vi "Set Controls State When Stopped.vi"(8 "error in (no error)":errorcluster, 11 "TS UI Data in":T1) -> (0 "error out":errorcluster)   [LabVIEW 2015]
uses:
  Type defs/TS UI Data.ctl
  Type defs/Nest cluster.ctl
panel:
  # "SCANNED DATA"
  # "ITAC DATA"
  # "DoIP DATA"
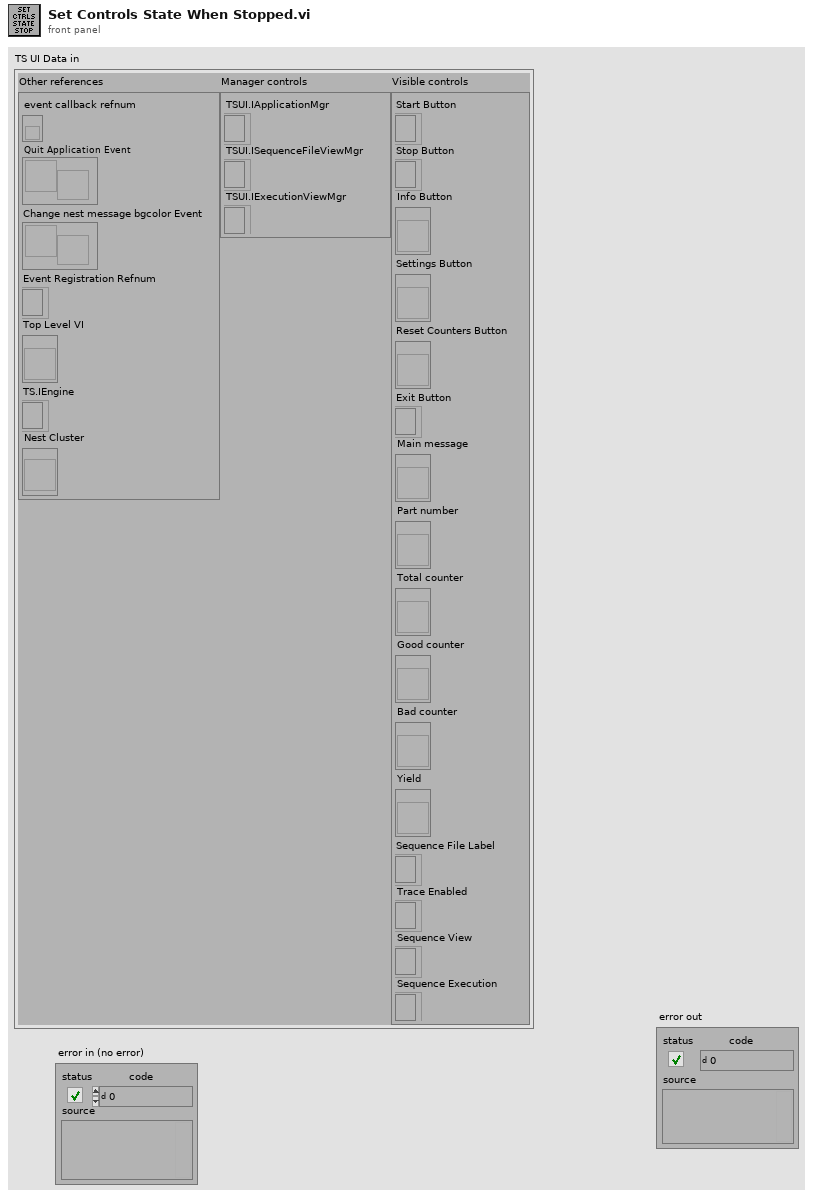
[diagram p1: front panel]
types:
  T1 = typedef "TS UI Data.ctl" = cluster{"Other references":cluster{"event callback refnum":refnum<k27>, "Quit Application Event":refnum<user-event>, "Change nest message bgcolor Event":refnum<user-event>, "event registration refnum":refnum<event-registration>, "Top Level VI":refnum<vi>, "TS.IEngine":refnum<k7>, "Nest Cluster":refnum<vi>}, "Manager controls":cluster{"TSUI.IApplicationMgr":refnum<k7>, "TSUI.ISequenceFileViewMgr":refnum<k7>, "TSUI.IExecutionViewMgr":refnum<k7>}, "Visible controls":cluster{"Start Button":refnum<k7>, "Stop Button":refnum<k7>, "Info Button":refnum<vi>, "Settings Button":refnum<vi>, "Reset Counters Button":refnum<vi>, "Exit Button":refnum<k7>, "Main message":refnum<vi>, "Part number":refnum<vi>, "Total counter":refnum<vi>, "Good counter":refnum<vi>, "Bad counter":refnum<vi>, "Yield":refnum<vi>, "Sequence File Label":refnum<k7>, "Trace Enabled":refnum<k7>, "Sequence View":refnum<k7>, "Sequence Execution":refnum<k7>}}
  T2 = enum8{"Enabled", "Disabled", "Disabled and Grayed Out"}
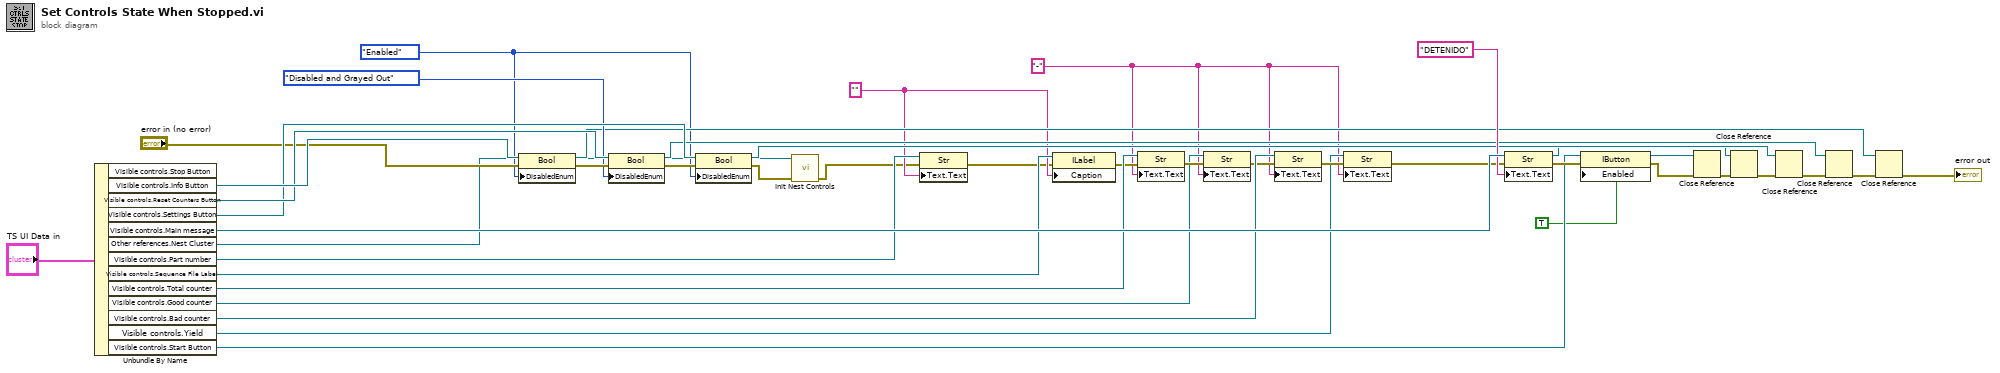
[diagram p0: block diagram]
diagram:
  w10 = "-" ("Text.Text")
  w12 = "" ("Text.Text")
  w25 = T2."Enabled" ("Disabled")
  n1 = Unbundle By Name("TS UI Data in") -> ("Visible controls.Info Button"=w42:refnum<vi>, "Visible controls.Reset Counters Button"=w41:refnum<vi>, "Visible controls.Settings Button"=w40:refnum<vi>, "Visible controls.Main message"=w36:refnum<vi>, "Other references.Nest Cluster"=w23:refnum<vi>, "Visible controls.Part number"=w22:refnum<vi>, "Visible controls.Sequence File Label"=w21:refnum<k7>, "Visible controls.Total counter"=w20:refnum<vi>, "Visible controls.Good counter"=w17:refnum<vi>, "Visible controls.Bad counter"=w16:refnum<vi>, "Visible controls.Yield"=w13:refnum<vi>, "Visible controls.Start Button"=w8:refnum<k7>)  [unwired: 1 out]
  n2 = property class="Bool"(reference=w42, error in="error in (no error)", "DisabledEnum"=w25) -> (reference out=w27:refnum<vi>, error out=w39:errorcluster)
  n3 = property class="Bool"(reference=w41, error in=w39, "DisabledEnum"=T2."Disabled and Grayed Out" ("Disabled")) -> (reference out=w29:refnum<vi>, error out=w38:errorcluster)
  n4 = property class="Bool"(reference=w40, error in=w38, "DisabledEnum"=w25) -> (reference out=w30:refnum<vi>, error out=w24:errorcluster)
  n5 = call "Init Nest Controls.vi"("error in (no error)"=w24, "Nest Cluster"=w23) -> ("error out"=w2:errorcluster)  [unwired: 9 in]
  n6 = property class="Str"(reference=w22, error in=w2, "Text.Text"=w12) -> (error out=w1:errorcluster)  [unwired: 1 out]
  n7 = property class="ILabel"(reference=w21, error in=w1, "Caption"=w12) -> (error out=w19:errorcluster)  [unwired: 1 out]
  n8 = property class="Str"(reference=w20, error in=w19, "Text.Text"=w10) -> (error out=w18:errorcluster)  [unwired: 1 out]
  n9 = property class="Str"(reference=w17, error in=w18, "Text.Text"=w10) -> (error out=w15:errorcluster)  [unwired: 1 out]
  n10 = property class="Str"(reference=w16, error in=w15, "Text.Text"=w10) -> (error out=w14:errorcluster)  [unwired: 1 out]
  n11 = property class="Str"(reference=w13, error in=w14, "Text.Text"=w10) -> (error out=w11:errorcluster)  [unwired: 1 out]
  n12 = property class="Str"(reference=w36, error in=w11, "Text.Text"="DETENIDO") -> (reference out=w3:refnum<vi>, error out=w9:errorcluster)
  n13 = property class="IButton"(reference=w8, error in=w9, "Enabled"=TRUE) -> (reference out=w4:refnum<k7>, error out=w5:errorcluster)
  n14 = Close Reference(reference=w4, error in (no error)=w5) -> (error out=w6:errorcluster)
  n15 = Close Reference(reference=w3, error in (no error)=w6) -> (error out=w32:errorcluster)
  n16 = Close Reference(reference=w30, error in (no error)=w32) -> (error out=w31:errorcluster)
  n17 = Close Reference(reference=w29, error in (no error)=w31) -> (error out=w28:errorcluster)
  n18 = Close Reference(reference=w27, error in (no error)=w28) -> (error out=→"error out":errorcluster)
